vi "Global References.vi"() -> ()   [LabVIEW 2020, in "RTAF.lvlib"]
uses:
  RTAF.lvlib
  Logger/API/Logger Actor API.lvclass
  Alarms Handler/API/Alarms Handler Actor API.lvclass
  Test/API/Test Actor API.lvclass
  System Status/API/System Status Actor API.lvclass
panel:
  in  "System Status":refnum<class "System Status Actor API.lvclass">
  in  "Test":refnum<class "Test Actor API.lvclass">
  in  "Alarms Handler":refnum<class "Alarms Handler Actor API.lvclass">
  in  "Logger":refnum<class "Logger Actor API.lvclass">
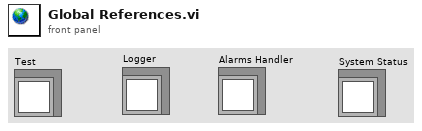
[diagram p1: front panel]
diagram:
